vi "BASE.Device.SetConfig.vi"(8 "error in (no error)":errorcluster, 10 "config":T1, 11 "BASE.Device in":refnum<class "BASE.Device.lvclass">) -> (0 "error out":errorcluster, 3 "BASE.Device out":refnum<class "BASE.Device.lvclass">)   [LabVIEW 2019, in "BASE.Device.lvlib" / "BASE.Device.lvclass"]
uses:
  BASE.Device.lvclass
  config--cluster.ctl
  BASE.Device.lvclass/BASE.Device.ctl
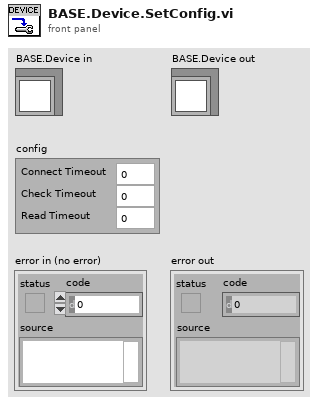
[diagram p1: front panel]
types:
  T1 = typedef "BASE.Device.lvlib/BASE.Device.lvclass/config--cluster.ctl" = cluster{"Connect Timeout":i32, "Check Timeout":i32, "Read Timeout":i32}
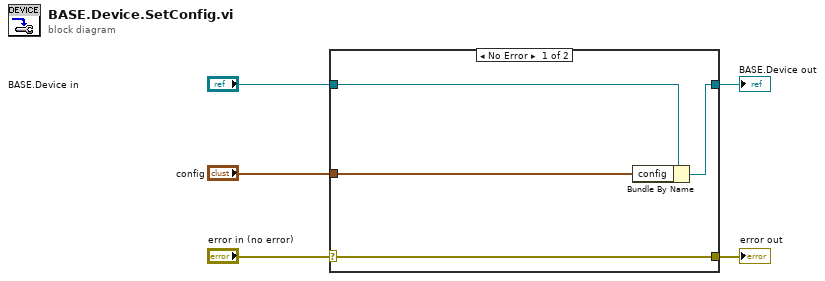
[diagram p0: block diagram]
diagram:
  n1 = case shown="No Error" "error in (no error)" {
    selector: "error in (no error)" -> [w9 w10]
    tunnel: [w9 w10] -> w4
    tunnel: [w7 w11] -> w2
    tunnel: "BASE.Device in" -> [w8 w11]
    tunnel: "config" -> [w6 _]
    frame No Error {
      n2 = Bundle By Name(cluster=w8, "config"=w6) -> (w7:refnum<class "BASE.Device.lvclass">)
    }
    frame Error {
    }
  }
  "error out" <- w4
  "BASE.Device out" <- w2
